vi "File Append.vi"(1 "file path":path=path "C:/Temp/TestFile.txt", 2 "text":string) -> ()   [LabVIEW 2021]
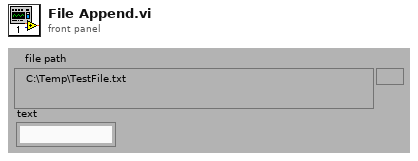
[diagram p1: front panel]
types:
  T1 = enum16{"open", "open or create", "create or replace", "create", "open (read only)"}
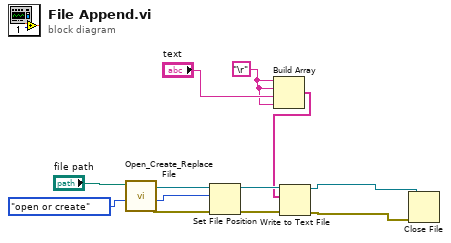
[diagram p0: block diagram]
diagram:
  w2 = "\r"
  n1 = call <vilib>:"Open_Create_Replace File.vi"("function (open:0)"=T1."open or create", "file path"="file path") -> ("error out"=w10:errorcluster, "file size (bytes)"=w8:i32, "refnum"=w9:refnum<file>)  [unwired: 6 in, 1 out]
  n2 = Set File Position(offset (in bytes) (0)=w8, refnum=w9, error in=w10) -> (refnum out=w7:refnum<file>, error out=w6:errorcluster)  [unwired: 1 in]
  n3 = Build Array(w2, w2, "text", w2) -> (w1:string[])
  n4 = Write to Text File(file (use dialog)=w7, text=w1, error in=w6) -> (refnum out=w4:refnum<file>, error out=w5:errorcluster)  [unwired: 1 in, 1 out]
  n5 = Close File(refnum=w4, error in=w5) -> ()  [unwired: 2 out]
